vi "Index Wertaenderung finden.vi"(8 "error in (no error)":errorcluster caption="Fehler (Eingang, kein Fehler)", 9 "neue Tabelle":string[][](table), 11 "alte Tabelle":string[][](table)) -> (0 "error out":errorcluster caption="Fehler (Ausgang)", 2 "Spalte":i32, 3 "Zeile":i32)   [LabVIEW 2020, in "Linearisierung v2.lvlib"]
uses:
  Linearisierung v2.lvlib
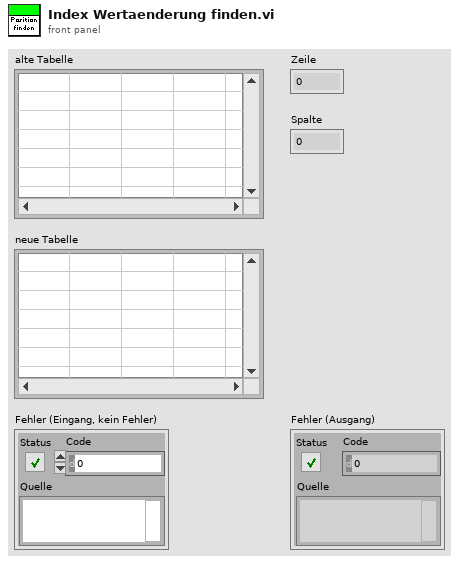
[diagram p1: front panel]
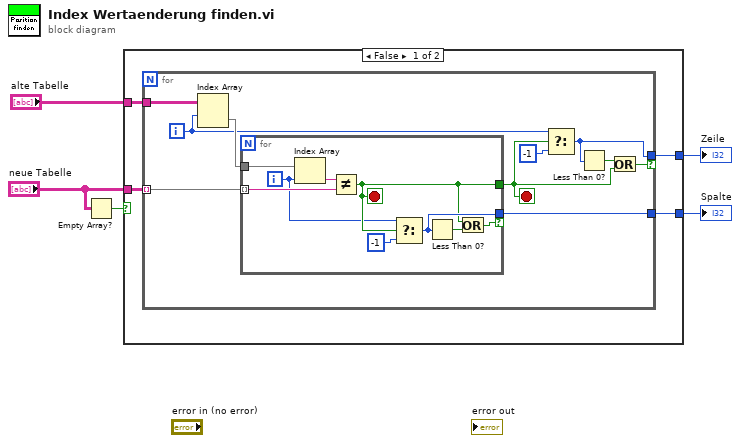
[diagram p0: block diagram]
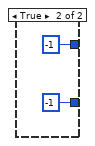
[diagram p2: hidden frame]
diagram:
  n1 = Empty Array?(array="neue Tabelle") -> (empty?=w1:bool)
  n2 = case shown="False" w1 {
    tunnel: "alte Tabelle" -> [w9 _]
    tunnel: [w8 -1] -> w4
    tunnel: [w7 -1] -> w3
    tunnel: "neue Tabelle" -> [w6 _]
    frame False {
      n3 = for {
        tunnel: w9 -> [w12]
        tunnel: w6 -> [w19] mode=indexing
        tunnel: [w18] -> w8
        tunnel: [w15] -> w7 if=w13
        i -> [w10]
        stop <- w14 stop-if-true
        n4 = Index Array(array=w12, index (row)=w10) -> (element=w11:string[])  [unwired: 1 in]
        n5 = for {
          tunnel: w19 -> [w28] mode=indexing
          tunnel: [w24] -> w14
          tunnel: [w26] -> w18 if=w23
          tunnel: w11 -> [w21]
          i -> [w20]
          stop <- w24 stop-if-true
          n6 = Index Array(array=w21, index=w20) -> (element=w22:string)
          n7 = Not Equal?(x=w22, y=w28) -> (x != y?=w24:bool)
          n8 = Select(t=w20, s=w24, f=-1) -> (s? t:f=w26:i32)
          n9 = Less Than 0?(x=w26) -> (x < 0?=w25:bool)
          n10 = Or(x=w24, y=w25) -> (x .or. y?=w23:bool)
        }
        n11 = Select(t=w10, s=w14, f=-1) -> (s? t:f=w15:i32)
        n12 = Less Than 0?(x=w15) -> (x < 0?=w16:bool)
        n13 = Or(x=w16, y=w14) -> (x .or. y?=w13:bool)
      }
    }
    frame True {
    }
  }
  "Spalte" <- w4
  "Zeile" <- w3
